vi "abc to dq conversion floating.vi"(5 "cos":sgl, 7 "sin":sgl, 9 "C":sgl, 10 "B":sgl, 11 "A":sgl) -> (0 "q":sgl format="%.2f", 3 "d":sgl format="%.2f")   [LabVIEW 2015]
uses:
  IP Cores/IP Cores - LabVIEW FPGA/Floating Point/Polymorphic subVIs/Multiply 00.vi
  IP Cores/IP Cores - LabVIEW FPGA/Floating Point/Polymorphic subVIs/Subtract 00.vi
  IP Cores/IP Cores - LabVIEW FPGA/Floating Point/Polymorphic subVIs/Add 00.vi
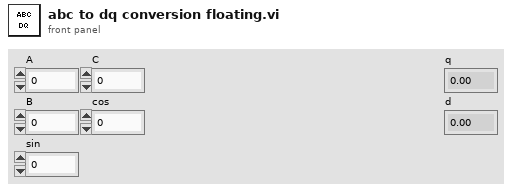
[diagram p1: front panel]
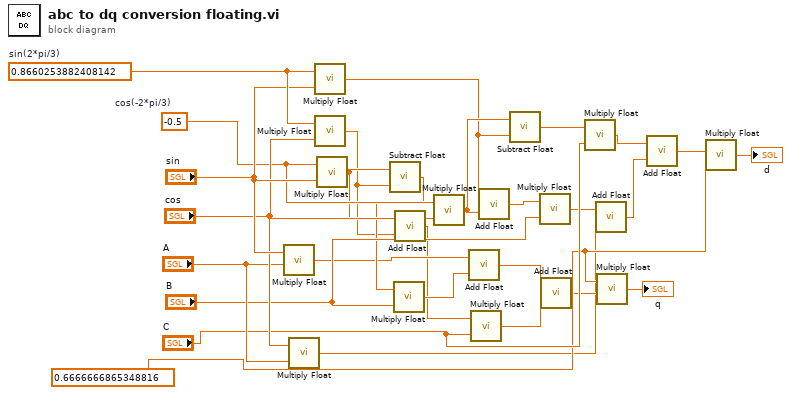
[diagram p0: block diagram]
diagram:
  w21 = sgl 0.6666667
  w25 = sgl -0.5  # cos(-2*pi/3)
  w28 = sgl 0.8660254  # sin(2*pi/3)
  n1 = call-poly "Multiply Float.vi"("y"="A", "x"="sin") -> ("x*y"=w19:sgl)
  n2 = call-poly "Multiply Float.vi"("y"="A", "x"="cos") -> ("x*y"=w8:sgl)
  n3 = call-poly "Multiply Float.vi"("y"="sin", "x"=w28) -> ("x*y"=w6:sgl)
  n4 = call-poly "Multiply Float.vi"("y"="cos", "x"=w28) -> ("x*y"=w16:sgl)
  n5 = call-poly "Multiply Float.vi"("y"="sin", "x"=w25) -> ("x*y"=w17:sgl)
  n6 = call-poly "Subtract Float.vi"("y"=w16, "x"=w17) -> ("x*y"=w20:sgl)
  n7 = call-poly "Multiply Float.vi"("y"="B", "x"=w20) -> ("x*y"=w18:sgl)
  n8 = call-poly "Add Float.vi"("y"=w16, "x"=w17) -> ("x+y"=w15:sgl)
  n9 = call-poly "Multiply Float.vi"("y"="cos", "x"=w25) -> ("x*y"=w7:sgl)
  n10 = call-poly "Add Float.vi"("y"=w18, "x"=w19) -> ("x+y"=w14:sgl)
  n11 = call-poly "Multiply Float.vi"("y"="C", "x"=w15) -> ("x*y"=w13:sgl)
  n12 = call-poly "Add Float.vi"("y"=w7, "x"=w6) -> ("x+y"=w10:sgl)
  n13 = call-poly "Subtract Float.vi"("y"=w6, "x"=w7) -> ("x*y"=w5:sgl)
  n14 = call-poly "Multiply Float.vi"("y"="B", "x"=w10) -> ("x*y"=w9:sgl)
  n15 = call-poly "Add Float.vi"("y"=w13, "x"=w14) -> ("x+y"=w12:sgl)
  n16 = call-poly "Multiply Float.vi"("y"="C", "x"=w5) -> ("x*y"=w4:sgl)
  n17 = call-poly "Add Float.vi"("y"=w8, "x"=w9) -> ("x+y"=w3:sgl)
  n18 = call-poly "Multiply Float.vi"("y"=w12, "x"=w21) -> ("x*y"=→"q":sgl)
  n19 = call-poly "Add Float.vi"("y"=w3, "x"=w4) -> ("x+y"=w2:sgl)
  n20 = call-poly "Multiply Float.vi"("y"=w21, "x"=w2) -> ("x*y"=→"d":sgl)
